vi "Lectura OSA.vi"() -> ()   [LabVIEW 2014]
panel:
  out "substring":string
  out "Espectro":cluster{dbl[], dbl[]}(graph)
  out "Respuesta OSA":string
  out "error out":errorcluster
  in  "Get data":bool
  in  "Send":bool
  out "?":bool
  in  "Sweep repeat":bool
  in  "Blank/Disp":bool=TRUE
  in  "?":bool
  in  "Stop":dbl=1570.0
  in  "Start":dbl=1470.0
  in  "Atributo":i32(listbox)
  in  "Trace":i32(listbox)
  in  "Preconfigurar":bool
  in  "Puerto":refnum<visa-resource-name>
  # "Sí"
  # "No"
  # "Span"
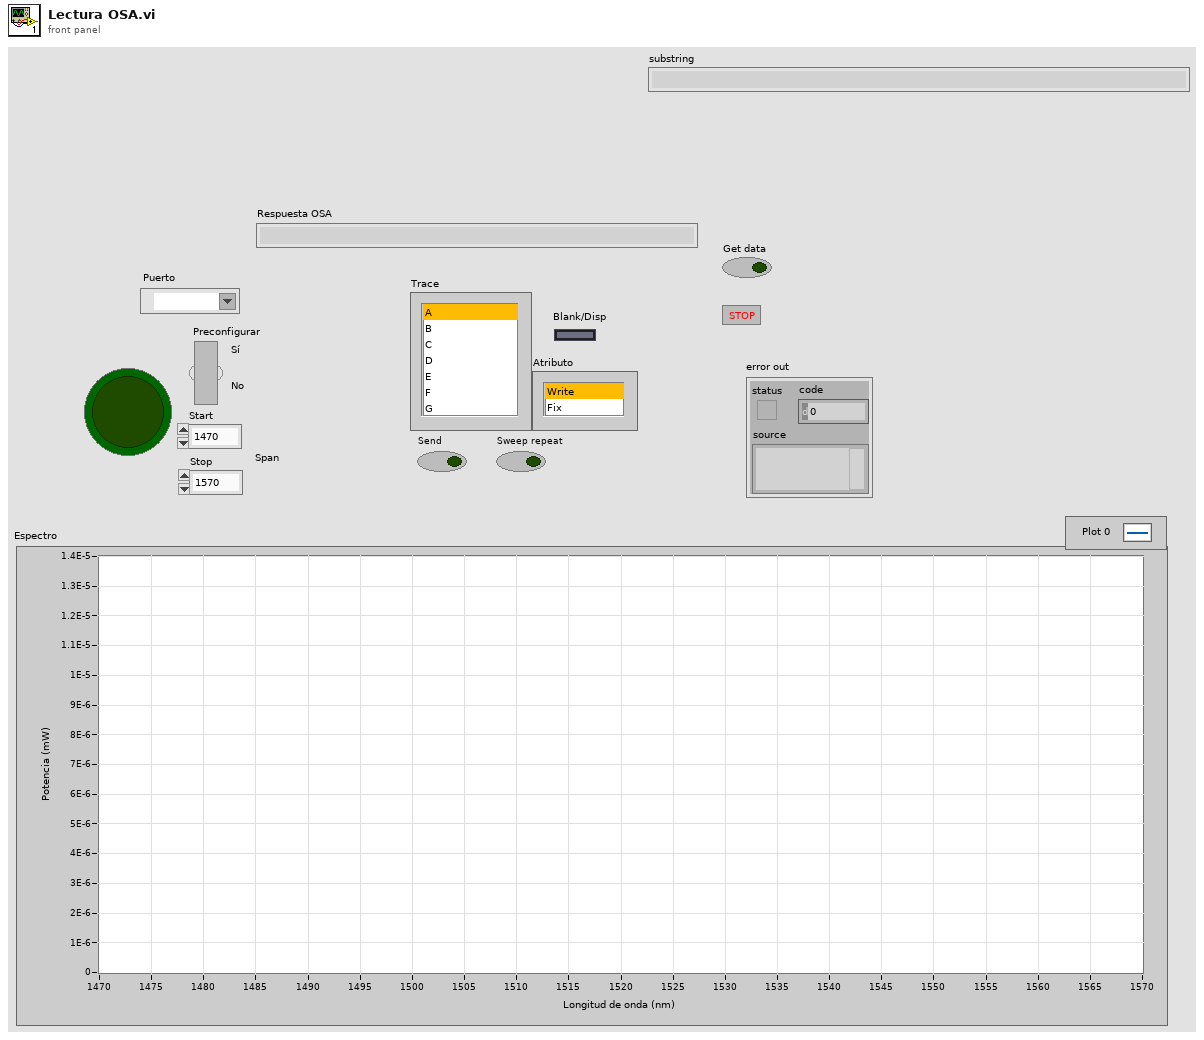
[diagram p1: front panel]
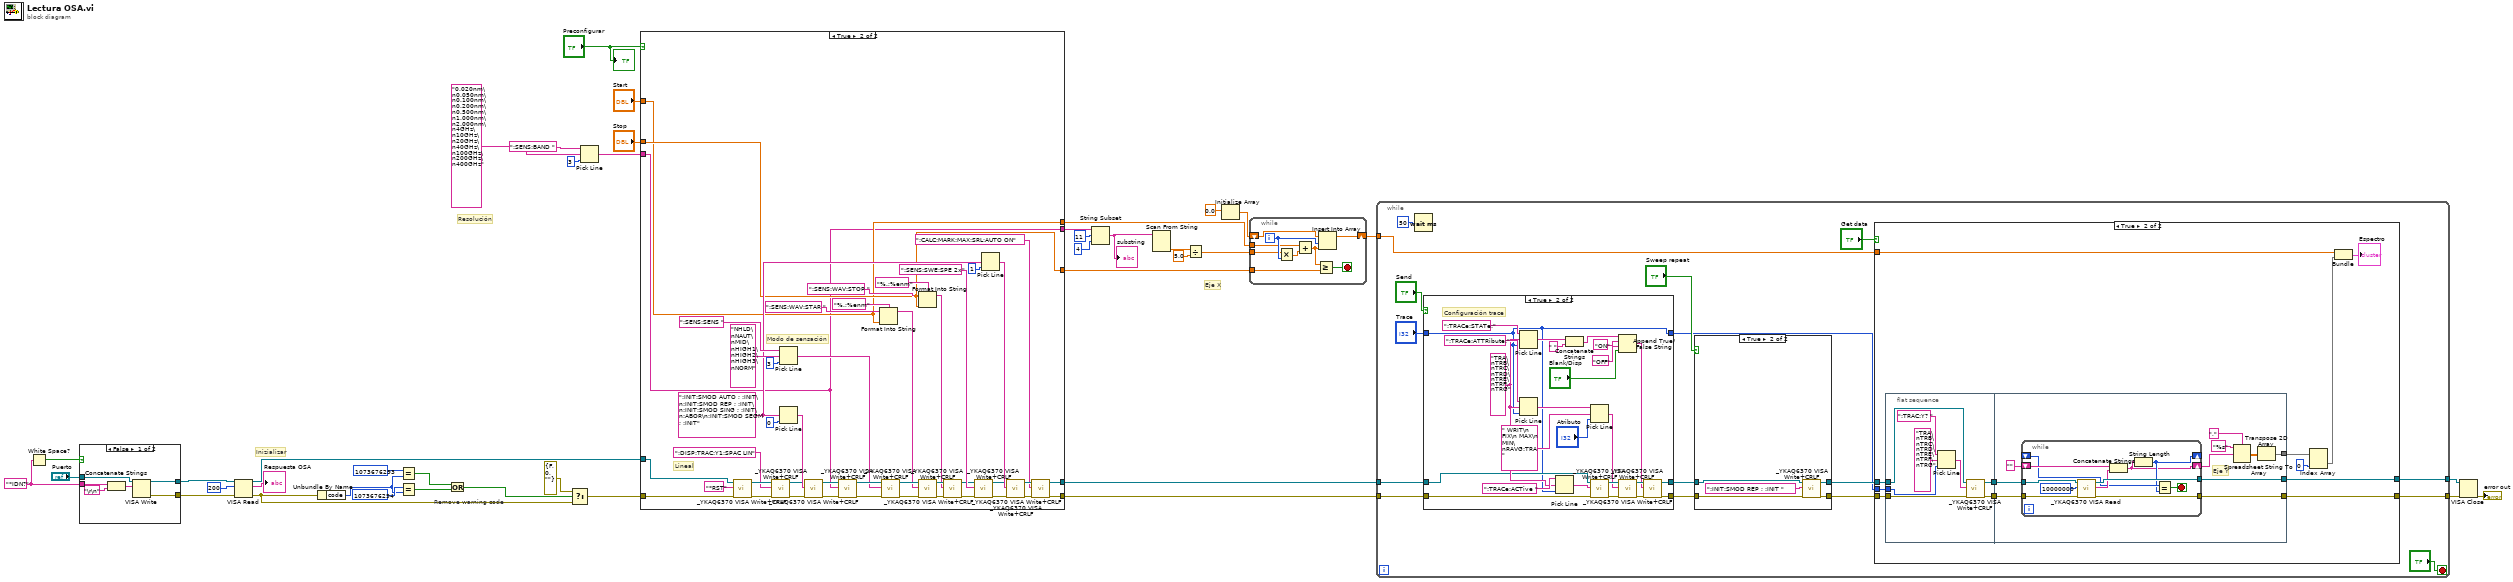
[diagram p0: block diagram]
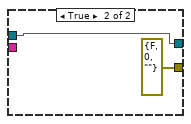
[diagram p6: hidden frame]
diagram:
  w39 = "*IDN?" ("Strings (empty)")
  # "Eje X"
  # "Resolución"
  # "Inizializar"
  # "Remove warning code"
  n1 = White Space?(1:w39) -> (0:w40:bool)
  n2 = case shown="False" w40 {
    tunnel: "Puerto" -> [w45 w49]
    tunnel: [w44 w49] -> w29
    tunnel: w39 -> [w43 _]
    tunnel: [w42 errorcluster {"status"=FALSE, "code"=0, "source"=""} ("error out")] -> w28
    frame False {
      n3 = Concatenate Strings(w43, "\r\n") -> (w46:string)
      n4 = VISA Write(VISA resource name=w45, write buffer=w46) -> (VISA resource name out=w44:refnum<visa-resource-name>, error out=w42:errorcluster)  [unwired: 1 in, 1 out]
    }
    frame True {
    }
  }
  n5 = VISA Read(VISA resource name=w29, byte count=u32 200 ("Byte Count (0)"), error in (no error)=w28) -> (VISA resource name out=w27:refnum<visa-resource-name>, read buffer=→"Respuesta OSA":string, error out=w36:errorcluster)  [unwired: 1 out]
  n6 = Unbundle By Name(w36) -> ("code"=w33:i32)
  n7 = Equal?(x=1073676293, y=w33) -> (x = y?=w32:bool)
  n8 = Equal?(x=1073676294, y=w33) -> (x = y?=w31:bool)
  n9 = Or(x=w32, y=w31) -> (x .or. y?=w30:bool)
  n10 = Select(t=errorcluster {"status"=FALSE, "code"=0, "source"=""}, s=w30, f=w36) -> (s? t:f=w26:errorcluster)
  n11 = Pick Line(string ("")=":SENS:BAND ", multi-line string="0.020nm\n0.050nm\n0.100nm\n0.200nm\n0.500nm\n1.000nm\n2.000nm\n4GHz\n10GHz\n20GHz\n40GHz\n100GHz\n200GHz\n400GHz", line index=3) -> (output string=w6:string)
  n12 = case shown="True" "Preconfigurar" {
    tunnel: w27 -> [w54 w97]
    tunnel: w26 -> [w53 w96]
    tunnel: [w54 w62] -> w25
    tunnel: [w53 w61] -> w24
    tunnel: [w50 w55] -> w19
    tunnel: [w52 w56] -> w14
    tunnel: [w51 w57] -> w13
    tunnel: "Stop" -> [w51 w57]
    tunnel: "Start" -> [w52 w56]
    tunnel: w6 -> [w50 w55]
    frame False {
    }
    frame True {
      w73 = ":INIT:SMOD AUTO ; :INIT\n:INIT:SMOD REP ; :INIT\n:INIT:SMOD SING ; :INIT\n:ABOR\n:INIT:SMOD SEGM ; :INIT"
      # "Lineal"
      # "Modo de sensación"
      n13 = call <instrlib>:"_YKAQ6370 VISA Write+CRLF.vi"("error in (no error)"=w96, "Strings (empty)"="*RST", "VISA resource name"=w97) -> ("error out"=w68:errorcluster, "VISA resource name out"=w69:refnum<visa-resource-name>)  [unwired: 7 in]
      n14 = call <instrlib>:"_YKAQ6370 VISA Write+CRLF.vi"("error in (no error)"=w68, "Strings (empty)"=":DISP:TRAC:Y1:SPAC LIN", "VISA resource name"=w69) -> ("error out"=w65:errorcluster, "VISA resource name out"=w66:refnum<visa-resource-name>)  [unwired: 7 in]
      n15 = Pick Line(string ("")=":SENS:SENS ", multi-line string="NHLD\nNAUT\nMID\nHIGH1\nHIGH2\nHIGH3\nNORM", line index=3) -> (output string=w89:string)
      n16 = Pick Line(multi-line string=w73, line index=0) -> (output string=w77:string)  [unwired: 1 in]
      n17 = call <instrlib>:"_YKAQ6370 VISA Write+CRLF.vi"("error in (no error)"=w65, "Strings (empty)"=w77, "VISA resource name"=w66) -> ("error out"=w78:errorcluster, "VISA resource name out"=w79:refnum<visa-resource-name>)  [unwired: 7 in]
      n18 = call <instrlib>:"_YKAQ6370 VISA Write+CRLF.vi"("error in (no error)"=w78, "Strings (empty)"=w55, "VISA resource name"=w79) -> ("error out"=w93:errorcluster, "VISA resource name out"=w92:refnum<visa-resource-name>)  [unwired: 7 in]
      n19 = Format Into String(format string="%.;%enm", initial string=":SENS:WAV:STAR ", w56) -> (resulting string=w83:string)  [unwired: 1 in, 1 out]
      n20 = call <instrlib>:"_YKAQ6370 VISA Write+CRLF.vi"("error in (no error)"=w93, "Strings (empty)"=w89, "VISA resource name"=w92) -> ("error out"=w94:errorcluster, "VISA resource name out"=w95:refnum<visa-resource-name>)  [unwired: 7 in]
      n21 = Format Into String(format string="%.;%enm", initial string=":SENS:WAV:STOP ", w57) -> (resulting string=w81:string)  [unwired: 1 in, 1 out]
      n22 = call <instrlib>:"_YKAQ6370 VISA Write+CRLF.vi"("error in (no error)"=w94, "Strings (empty)"=w83, "VISA resource name"=w95) -> ("error out"=w86:errorcluster, "VISA resource name out"=w87:refnum<visa-resource-name>)  [unwired: 7 in]
      n23 = call <instrlib>:"_YKAQ6370 VISA Write+CRLF.vi"("error in (no error)"=w86, "Strings (empty)"=w81, "VISA resource name"=w87) -> ("error out"=w63:errorcluster, "VISA resource name out"=w64:refnum<visa-resource-name>)  [unwired: 7 in]
      n24 = call <instrlib>:"_YKAQ6370 VISA Write+CRLF.vi"("error in (no error)"=w63, "Strings (empty)"=":SENS:SWE:SPE 2x", "VISA resource name"=w64) -> ("error out"=w71:errorcluster, "VISA resource name out"=w72:refnum<visa-resource-name>)  [unwired: 7 in]
      n25 = Pick Line(multi-line string=w73, line index=1) -> (output string=w74:string)  [unwired: 1 in]
      n26 = call <instrlib>:"_YKAQ6370 VISA Write+CRLF.vi"("error in (no error)"=w71, "Strings (empty)"=w74, "VISA resource name"=w72) -> ("error out"=w59:errorcluster, "VISA resource name out"=w60:refnum<visa-resource-name>)  [unwired: 7 in]
      n27 = call <instrlib>:"_YKAQ6370 VISA Write+CRLF.vi"("error in (no error)"=w59, "Strings (empty)"=":CALC:MARK:MAX:SRL:AUTO ON", "VISA resource name"=w60) -> ("error out"=w61:errorcluster, "VISA resource name out"=w62:refnum<visa-resource-name>)  [unwired: 7 in]
    }
  }
  n28 = String Subset(string=w19, offset (0)=11, length (rest)=4 ("length (rest)")) -> (substring=w17:string)
  "substring" <- w17
  n29 = Scan From String(input string=w17) -> (output 1=w5:dbl)  [unwired: 4 in, 3 out]
  n30 = Divide(x=w5, y=5.0) -> (x/y=w4:dbl)
  n31 = Initialize Array(0.0 ("element")) -> (w16:dbl[])  [unwired: 1 in]
  n32 = while {
    shift-right: [w106] -> w2
    shift-left: w16 -> [w107]
    tunnel: w14 -> [w102]
    tunnel: w4 -> [w104]
    tunnel: w13 -> [w100]
    i -> [w105]
    stop <- w99 stop-if-true
    n33 = Multiply(x=w104, y=w105) -> (x*y=w103:dbl)
    n34 = Add(x=w102, y=w103) -> (x+y=w101:dbl)
    n35 = Greater Or Equal?(x=w101, y=w100) -> (x >= y?=w99:bool)
    n36 = Insert Into Array(array=w107, index=w105, new element=w101) -> (w106:dbl[])
  }
  n37 = while {
    tunnel: w25 -> [w123]
    tunnel: w24 -> [w122]
    tunnel: [w112] -> w1
    tunnel: [w111] -> w21
    tunnel: w2 -> [w110]
    stop <- "?" stop-if-true
    n38 = Wait (ms)(milliseconds to wait=u32 50) -> ()  [unwired: 1 out]
    n39 = case shown="True" "Send" {
      tunnel: w123 -> [w176 w182]
      tunnel: w122 -> [w175 w181]
      tunnel: [w176 w180] -> w120
      tunnel: [w175 w179] -> w119
      tunnel: [w174 w177] -> w109
      tunnel: "Trace" -> [w174 w177]
      frame False {
      }
      frame True {
        w184 = "TRA\nTRB\nTRC\nTRD\nTRE\nTRF\nTRG"
        # "Configuración trace"
        n40 = Pick Line(string ("")=":TRACe:STATe:", multi-line string=w184, line index=w177) -> (output string=w185:string)
        n41 = Pick Line(string ("")=":TRACe:ATTRibute:", multi-line string=w184, line index=w177) -> (output string=w190:string)
        n42 = Pick Line(string ("")=":TRACe:ACTive ", multi-line string=w184, line index=w177) -> (output string=w186:string)
        n43 = Concatenate Strings(w185, " " ("string")) -> (w188:string)
        n44 = Pick Line(string ("")=w190, multi-line string=" WRIT\n FIX\n MAX\n MIN\nRAVG:TRA ", line index="Atributo") -> (output string=w189:string)
        n45 = call <instrlib>:"_YKAQ6370 VISA Write+CRLF.vi"("error in (no error)"=w181, "Strings (empty)"=w186, "VISA resource name"=w182) -> ("error out"=w198:errorcluster, "VISA resource name out"=w197:refnum<visa-resource-name>)  [unwired: 7 in]
        n46 = Append True/False String(1:"Blank/Disp", 2:"OFF", 3:"ON", 4:w188) -> (0:w194:string)
        n47 = call <instrlib>:"_YKAQ6370 VISA Write+CRLF.vi"("error in (no error)"=w198, "Strings (empty)"=w189, "VISA resource name"=w197) -> ("error out"=w195:errorcluster, "VISA resource name out"=w196:refnum<visa-resource-name>)  [unwired: 7 in]
        n48 = call <instrlib>:"_YKAQ6370 VISA Write+CRLF.vi"("error in (no error)"=w195, "Strings (empty)"=w194, "VISA resource name"=w196) -> ("error out"=w179:errorcluster, "VISA resource name out"=w180:refnum<visa-resource-name>)  [unwired: 7 in]
      }
    }
    n49 = case shown="True" "Sweep repeat" {
      tunnel: w120 -> [w168 w173]
      tunnel: w119 -> [w167 w172]
      tunnel: [w168 w170] -> w115
      tunnel: [w167 w169] -> w114
      frame False {
      }
      frame True {
        n50 = call <instrlib>:"_YKAQ6370 VISA Write+CRLF.vi"("error in (no error)"=w172, "Strings (empty)"=":INIT:SMOD REP ; :INIT ", "VISA resource name"=w173) -> ("error out"=w169:errorcluster, "VISA resource name out"=w170:refnum<visa-resource-name>)  [unwired: 7 in]
      }
    }
    n51 = case shown="True" "Get data" {
      tunnel: w115 -> [w124 w137]
      tunnel: w114 -> [w125 w136]
      tunnel: [w125 w132] -> w112
      tunnel: [w124 w133] -> w111
      tunnel: w110 -> [_ w128]
      tunnel: w109 -> [_ w126]
      frame False {
      }
      frame True {
        n52 = flat-sequence {
          tunnel: w137 -> [w145]
          tunnel: w136 -> [w144]
          tunnel: [w143] -> w135
          tunnel: [w142] -> w134
          tunnel: w126 -> [w138]
          tunnel: w135 -> [w155]
          tunnel: w134 -> [w154]
          tunnel: [w148] -> w131
          tunnel: [w147] -> w133
          tunnel: [w146] -> w132
          frame #0 {
            n53 = Pick Line(string ("")=":TRAC:Y? " ("Strings (empty)"), multi-line string="TRA\nTRB\nTRC\nTRD\nTRE\nTRF\nTRG", line index=w138) -> (output string=w139:string)
            n54 = call <instrlib>:"_YKAQ6370 VISA Write+CRLF.vi"("error in (no error)"=w144, "Strings (empty)"=w139, "VISA resource name"=w145) -> ("error out"=w142:errorcluster, "VISA resource name out"=w143:refnum<visa-resource-name>)  [unwired: 7 in]
          }
          frame #1 {
            # "Eje Y"
            n55 = while {
              tunnel: w155 -> [w165]
              tunnel: w154 -> [w164]
              tunnel: [w163] -> w147
              tunnel: [w162] -> w146
              shift-right: [w156] -> w152
              shift-left: "" -> [w161]
              shift-right: [w158] -> _
              shift-left: _ -> [w159]
              stop <- w157 stop-if-true
              n56 = call <instrlib>:"_YKAQ6370 VISA Read.vi"("error in (no error)"=w164, "Byte Count (0)"=u32 10000000, "VISA resource name"=w165) -> ("error out"=w162:errorcluster, "Read Data"=w160:string, "VISA resource name out"=w163:refnum<visa-resource-name>)  [unwired: 5 in, 1 out]
              n57 = Concatenate Strings(w161, w160) -> (w156:string)
              n58 = String Length(string=w156) -> (length=w158:i32)
              n59 = Equal?(x=w159, y=w158) -> (x = y?=w157:bool)
            }
            n60 = Spreadsheet String To Array(delimiter (Tab)=",", format string="%s", spreadsheet string=w152) -> (array=w149:dbl[][])  [unwired: 1 in]
            n61 = Transpose 2D Array(2D array=w149) -> (transposed array=w148:dbl[][])
          }
        }
        n62 = Index Array(array=w131, index (col)=0 ("disabled index (col)")) -> (element=w129:dbl[])  [unwired: 1 in]
        n63 = Bundle(w128, w129) -> (→"Espectro":cluster{dbl[], dbl[]})  [unwired: 1 in]
      }
    }
  }
  n64 = VISA Close(VISA resource name=w21, error in (no error)=w1) -> (error out=→"error out":errorcluster)
  "?" <- "Preconfigurar"
